vi "Analyze Data.vi"(8 "error in":errorcluster, 11 "PAS in":refnum<class "PAS.lvclass">) -> (0 "error out":errorcluster, 3 "PAS out":refnum<class "PAS.lvclass">)   [LabVIEW 2015, in "PAS.lvclass"]
doc: "This is the core routine for PAS microphone data analysis. Here, the microphone data is retrieved from each of the cells. In both cases, the time domain signal will be transformed to the frequency domain. If the speaker is on (<B>Spk Pos</B> == TRUE), then the frequency domain signal will be squared to obtain the power and a Lorentzian will be fit to the data to retrieve the resonant characteristics of the cell. If the speaker is off (<B>Spk Pos</B> == FALSE), then the amplitude will be used to calculate the integrated area of the signal. In every case, the implementation has the ability to decimate the data for transmission of the waveforms over a network line."
uses:
  PAS.lvclass
  PAS.lvclass/PAS.ctl
  <vilib>/Analysis/4window.llb/windowTd.ctl
  Read Chirp.vi
  Get Speaker State.vi
  Data/Main/Write drive.vi
  Data/Main/Read CellData.vi
  Data/Main/Read filter.vi
  Cell/Read extParams.vi
  Data/Cell/Read timeData.vi
  Data/Cell/Read lasDiodeData.vi
  <vilib>/measure/maspectr.llb/FFT Spectrum (Mag-Phase) for 1 Chan.vi
  Data/Cell/Get Integrated Area.vi
  Data/Cell/Read derived.vi
  Data/Cell/Write lasDiodeData.vi
  Data/Cell/Write derived.vi
  Data/Cell/PAS Cell Data.lvclass
  <vilib>/Analysis/NI_AALPro.lvlib
  Data/Main/PAS Data.lvclass
  Instrument/Instrument.lvclass
  <vilib>/measure/NI_MAPro.lvlib
  Cell/PAS Cell.lvclass
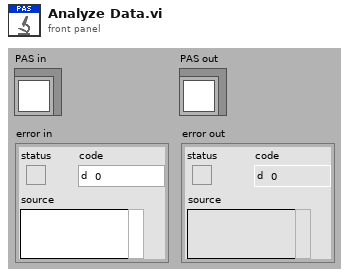
[diagram p1: front panel]
types:
  T1 = typedef "NI_AALPro.lvlib/windowTd.ctl" = u32
  T2 = cluster{"f0":sgl, "IA":sgl, "Q":sgl, "max":dbl[], "deltaPhi":dbl, "tau":dbl, "noiseLim":dbl, "ext":dbl}
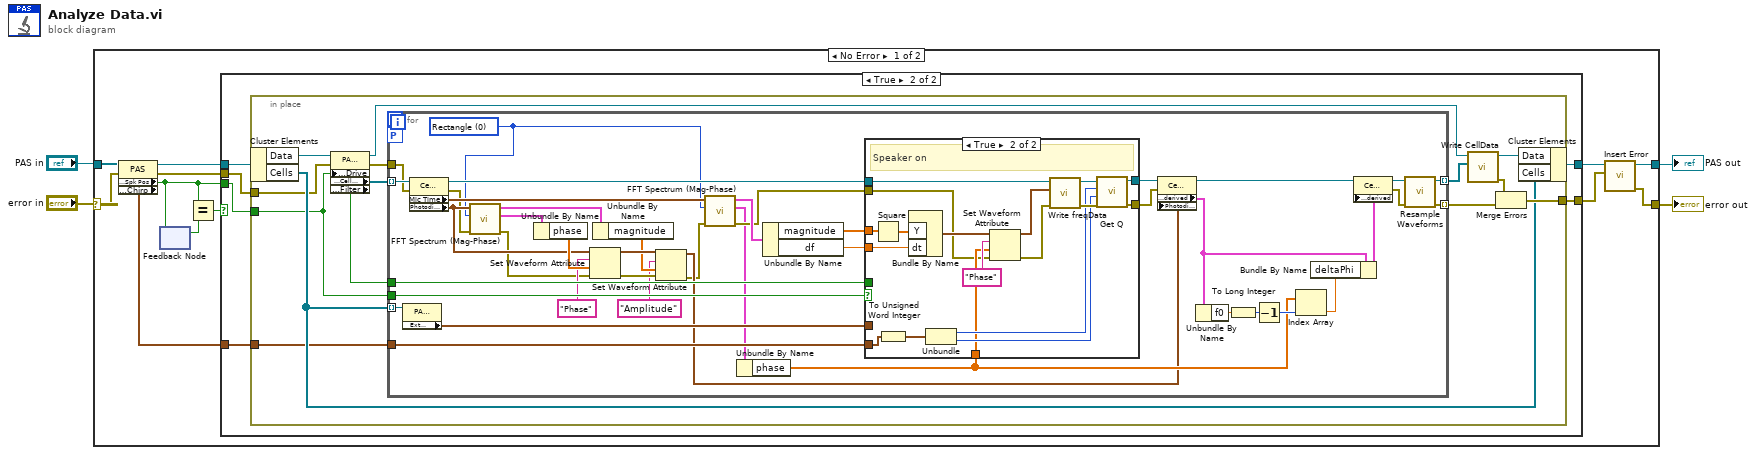
[diagram p0: block diagram]
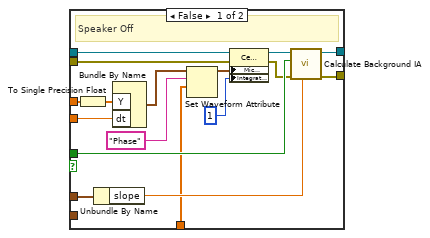
[diagram p3: hidden frame]
diagram:
  n1 = case shown="No Error" "error in" {
    selector: "error in" -> [w10 w117]
    tunnel: [w14 w117] -> w1
    tunnel: [w15 w116] -> w2
    tunnel: "PAS in" -> [w13 w116]
    frame No Error {
      n2 = property class="PAS"(reference=w13, error in=w10) -> (reference out=w12:refnum<class "PAS.lvclass">, error out=w11:errorcluster, "Data Access:Spk Pos"=w5:bool, "Data Access:Chirp"=w9:cluster{"f_center":dbl, "bandwidth":dbl})
      n3 = feedback-in #1(w5) -> ()
      n4 = feedback #1() -> (w6:bool)  [unwired: 1 in]
      n5 = Equal?(x=w5, y=w6) -> (x = y?=w7:bool)
      n6 = case shown="True" w7 {
        tunnel: [w18 w24] -> w16
        tunnel: w12 -> [w18 w23]
        tunnel: w11 -> [w17 w22]
        tunnel: w5 -> [_ w21]
        tunnel: w9 -> [_ w19]
        tunnel: [w17 w20] -> w8
        frame False {
        }
        frame True {
          n7 = in-place {
            in-place-border: [w35] -> w20
            in-place-border: w22 -> [w26]
            in-place-border: w21 -> [w30]
            in-place-border: w19 -> [w32]
            n8 = in-place-cluster #2(w23) -> ("Data"=w31:refnum<class "PAS Data.lvclass">, "Cells"=w33:refnum<class "PAS Cell.lvclass">[])
            n9 = property class="PAS Data"(reference=w31, error in=w26, "Data Access:Drive"=w30) -> (reference out=w28:refnum<class "PAS Data.lvclass">, error out=w27:errorcluster, "Data Access:Cell Data"=w29:refnum<class "PAS Cell Data.lvclass">[], "Data Access:Filter"=w25:bool)
            n10 = for {
              tunnel: w29 -> [w58] mode=indexing
              tunnel: [w80] -> w38 mode=indexing
              tunnel: [w79] -> w37 mode=indexing
              workers-P: _ -> [_]
              tunnel: w30 -> [w74]
              tunnel: w27 -> [w48]
              tunnel: w33 -> [w73] mode=indexing
              tunnel: w32 -> [w71]
              tunnel: w25 -> [w70]
              w39 = T1 0 items=["Rectangle"=0, "Hanning"=1, "Hamming"=2, "Blackman-Harris"=3, "Exact Blackman"=4, "Blackman"=5, "Flat Top"=6, "4 Term B-Harris "=7, "7 Term B-Harris"=8, "Low Sidelobe"=9, "Blackman Nuttall"=11, "Triangle"=30, "Bartlett-Hanning"=31, "Bohman"=32, "Parzen"=33, "Welch"=34, "Kaiser"=60, "Dolph-Chebyshev"=61, "Gaussian"=62] ("window")
              n11 = property class="PAS Cell"(reference=w73) -> ("Ext Params"=w72:cluster{"slope":sgl, "zero":sgl})  [unwired: 1 in, 2 out]
              n12 = property class="Cell Data"(reference=w58, error in=w48) -> (reference out=w57:refnum<class "PAS Cell Data.lvclass">, error out=w49:errorcluster, "Mic Time"=w56:waveform(i16), "Photodiode"=w53:waveform(i16))
              n13 = call-poly <vilib>:"FFT Spectrum (Mag-Phase).vi"("error in (no error)"=w49, "window"=w39, "time signal"=w53) -> ("error out"=w47:errorcluster, "phase"=w55:cluster{"f0":dbl, "df":dbl, "phase":dbl[]}, "magnitude"=w44:cluster{"f0":dbl, "df":dbl, "magnitude":dbl[]})  [unwired: 4 in, 2 out]
              n14 = Unbundle By Name(w55) -> ("phase"=w54:dbl[])
              n15 = Set Waveform Attribute(4:w47, 5:w54, 6:"Phase" ("name"), 7:w53) -> (0:w45:errorcluster, 3:w46:waveform(i16))  [unwired: 1 out]
              n16 = Unbundle By Name(w44) -> ("magnitude"=w43:dbl[])
              n17 = Set Waveform Attribute(4:w45, 5:w43, 6:"Amplitude" ("name"), 7:w46) -> (0:w40:errorcluster, 3:w41:waveform(i16))  [unwired: 1 out]
              n18 = call-poly <vilib>:"FFT Spectrum (Mag-Phase).vi"("error in (no error)"=w40, "window"=w39, "time signal"=w56) -> ("error out"=w77:errorcluster, "phase"=w69:cluster{"f0":dbl, "df":dbl, "phase":dbl[]}, "magnitude"=w78:cluster{"f0":dbl, "df":dbl, "magnitude":dbl[]})  [unwired: 4 in, 2 out]
              n19 = Unbundle By Name(w69) -> ("phase"=w59:dbl[])
              n20 = Unbundle By Name(w78) -> ("magnitude"=w76:dbl[], "df"=w75:dbl)
              n21 = case shown="True" w74 {
                tunnel: w57 -> [w89 w110]
                tunnel: w77 -> [w87 w99]
                tunnel: [w95 w115] -> w50
                tunnel: [w96 w114] -> w51
                tunnel: w76 -> [w91 w109]
                tunnel: w75 -> [w97 w111]
                tunnel: w72 -> [w93 _]
                tunnel: w71 -> [_ w105]
                tunnel: w70 -> [w94 _]
                tunnel: w59 -> [w81 w100]
                frame False {
                  # "Speaker Off"
                  n22 = To Single Precision Float(number=w91) -> (single precision float=w90:sgl[])
                  n23 = Unbundle By Name(w93) -> ("slope"=w92:sgl)
                  n24 = Bundle By Name("Y"=w90, "dt"=w97) -> (w84:waveform(sgl))  [unwired: 1 out]
                  n25 = Set Waveform Attribute(5:w81, 6:"Phase" ("name"), 7:w84) -> (3:w83:waveform(sgl))  [unwired: 1 in, 2 out]
                  n26 = property class="Cell Data"(reference=w89, error in=w87, "Mic Frequency"=w83, "Integrated Area"=1) -> (reference out=w85:refnum<class "PAS Cell Data.lvclass">, error out=w86:errorcluster)
                  n27 = call "Calculate Background IA.vi"("Slope"=w92, "error in"=w86, "Filter"=w94, "Cell Data in"=w85) -> ("error out"=w95:errorcluster, "Cell Data out"=w96:refnum<class "PAS Cell Data.lvclass">)  [unwired: 6 in]
                }
                frame True {
                  # "Speaker on"
                  n28 = Square(x=w109) -> (x^2=w108:dbl[])
                  n29 = To Unsigned Word Integer(number=w105) -> (unsigned 16bit integer=w104:cluster{"f_center":u16, "bandwidth":u16})
                  n30 = Bundle By Name("Y"=w108, "dt"=w111) -> (w102:waveform(dbl))  [unwired: 1 out]
                  n31 = Unbundle(w104) -> ("f_center"=w107:u16, "bandwidth"=w106:u16)
                  n32 = Set Waveform Attribute(4:w99, 5:w100, 6:"Phase" ("name"), 7:w102) -> (0:w98:errorcluster, 3:w101:waveform(dbl))  [unwired: 1 out]
                  n33 = call "Write freqData.vi"("error in (no error)"=w98, "freqData"=w101, "PAS Cell Data in"=w110) -> ("error out"=w112:errorcluster, "PAS Cell Data out"=w113:refnum<class "PAS Cell Data.lvclass">)  [unwired: 7 in]
                  n34 = call "Get Q.vi"("error in"=w112, "Bandwidth"=w106, "f_center"=w107, "PAS Cell Data in"=w113) -> ("error out"=w115:errorcluster, "PAS Cell Data out"=w114:refnum<class "PAS Cell Data.lvclass">)  [unwired: 6 in]
                }
              }
              n35 = property class="Cell Data"(reference=w51, error in=w50, "Photodiode"=w41) -> (reference out=w68:refnum<class "PAS Cell Data.lvclass">, "Data Access:derived"=w65:T2)  [unwired: 1 out]
              n36 = Unbundle By Name(w65) -> ("f0"=w63:sgl)
              n37 = To Long Integer(number=w63) -> (32bit integer=w62:i32)
              n38 = Decrement(x=w62) -> (x-1=w61:i32)
              n39 = Index Array(array=w59, index=w61) -> (element=w60:dbl)
              n40 = Bundle By Name(cluster=w65, "deltaPhi"=w60) -> (w64:T2)
              n41 = property class="Cell Data"(reference=w68, "Data Access:derived"=w64) -> (reference out=w67:refnum<class "PAS Cell Data.lvclass">, error out=w66:errorcluster)  [unwired: 1 in]
              n42 = call "Resample Waveforms.vi"("error in"=w66, "PAS Cell Data in"=w67) -> ("error out"=w79:errorcluster, "PAS Cell Data out"=w80:refnum<class "PAS Cell Data.lvclass">)  [unwired: 8 in]
            }
            n43 = call "Write CellData.vi"("CellData"=w38, "PAS Data in"=w28) -> ("error out"=w36:errorcluster, "PAS Data out"=w34:refnum<class "PAS Data.lvclass">)  [unwired: 8 in]
            n44 = Merge Errors(w36, w37) -> (w35:errorcluster)
            n45 = in-place-cluster #2("Data"=w34, "Cells"=w33) -> (w24:refnum<class "PAS.lvclass">)
          }
        }
      }
      n46 = call "Insert Error.vi"("err"=w8, "Instrument in"=w16) -> ("error out"=w14:errorcluster, "Instrument out"=w15:refnum<class "PAS.lvclass">)  [unwired: 7 in, 1 out]
    }
    frame Error {
    }
  }
  "error out" <- w1
  "PAS out" <- w2
